vi "Set Up Dialog - Water Quality Lab.vi"() -> ()   [LabVIEW 2012]
panel:
  in  "CTSN Set Up":bool
  in  "CMN Set Up":bool
  in  "D02 Set Up":bool
  in  "pH Set Up":bool
  out "Calibration Instructions":string="This Lab is designed to use four different sensors (DO2N-200E, PHN-100, CMN-100, and CTSN-100) one at a time to measure the qualities of a water sample. "
  # "iWorx - Water Quality Lab - Set Up"
  # "pH Sensor (PHN - 100)"
  # "Dissolved Oxygen (D02N - 300)"
  # "Conductivity sensor (CMN-100)"
  # "Colorimeter (CTSN - 100)"
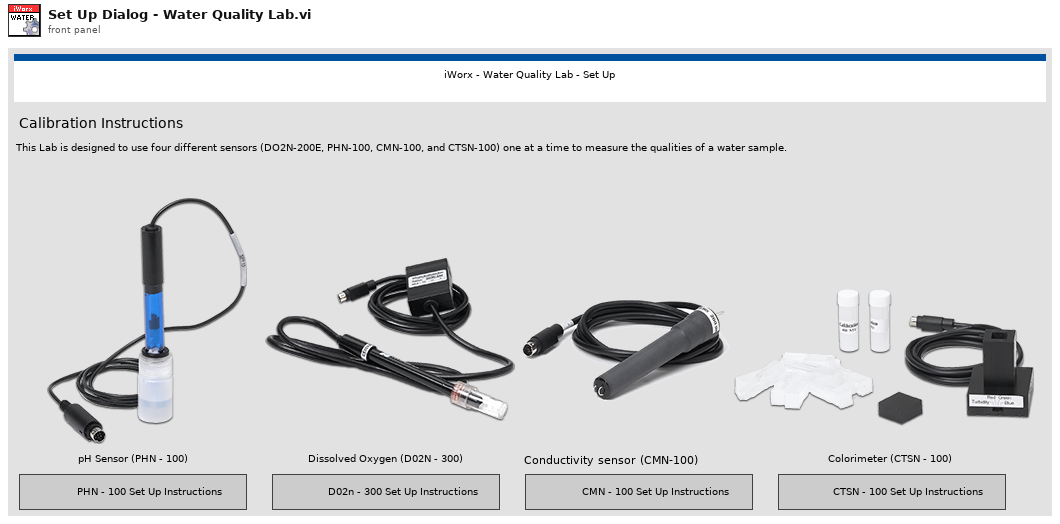
[diagram p1: front panel]
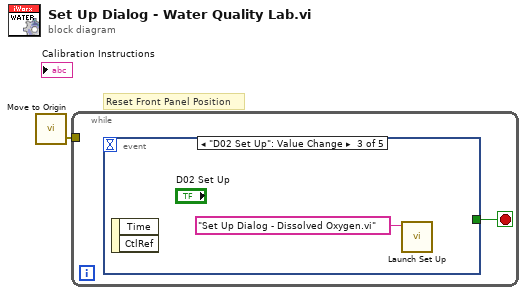
[diagram p0: block diagram]
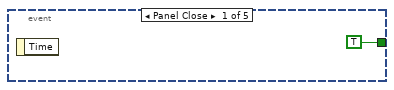
[diagram p2: hidden frame]
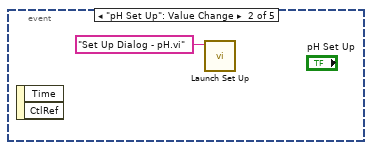
[diagram p3: hidden frame]
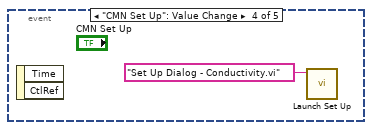
[diagram p4: hidden frame]
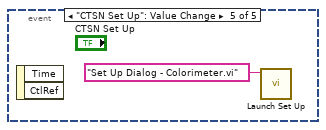
[diagram p5: hidden frame]
diagram:
  # "Reset Front Panel Position"
  n1 = call "Move to Origin.vi"() -> ("Error Out"=w1:errorcluster)  [unwired: 3 in]
  n2 = while {
    tunnel: w1 -> [_]
    stop <- w2 stop-if-true
    n3 = event shown="[2] \"D02 Set Up\": Value Change" {
      selector: _ -> [_ _ _ _ _]
      dyn-events: _ -> [_ _ _ _ _]
      timeout: _ -> [_ _ _ _ _]
      tunnel: [TRUE _ _ _ _] -> w2
      event Panel Close {
        n4 = event-data() -> ()  [unwired: 1 in, 1 out]
      }
      event "pH Set Up": Value Change {
        n5 = event-data() -> ()  [unwired: 1 in, 2 out]
        n6 = call "Launch Set Up.vi"("name or relative path"="Set Up Dialog - pH.vi") -> ()  [unwired: 9 in, 2 out]
      }
      event "D02 Set Up": Value Change {
        n7 = event-data() -> ()  [unwired: 1 in, 2 out]
        n8 = call "Launch Set Up.vi"("name or relative path"="Set Up Dialog - Dissolved Oxygen.vi") -> ()  [unwired: 9 in, 2 out]
      }
      event "CMN Set Up": Value Change {
        n9 = event-data() -> ()  [unwired: 1 in, 2 out]
        n10 = call "Launch Set Up.vi"("name or relative path"="Set Up Dialog - Conductivity.vi") -> ()  [unwired: 9 in, 2 out]
      }
      event "CTSN Set Up": Value Change {
        n11 = event-data() -> ()  [unwired: 1 in, 2 out]
        n12 = call "Launch Set Up.vi"("name or relative path"="Set Up Dialog - Colorimeter.vi") -> ()  [unwired: 9 in, 2 out]
      }
    }
  }
